vi "aft_xmpl_Shaker Simulation.vi"(8 "error in (no error)":errorcluster, 11 "drive signal":dbl[](array[numeric])) -> (0 "error out":errorcluster, 3 "shaker output":dbl[](array[numeric]))   [LabVIEW 2023]
uses:
  <vilib>/Analysis/3filter.llb/FIR Filter (DBL).vi
  <vilib>/Analysis/NI_AALBase.lvlib
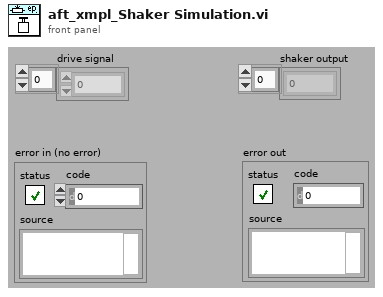
[diagram p1: front panel]
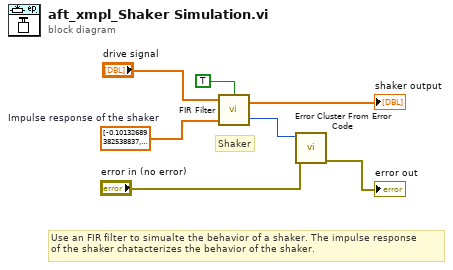
[diagram p0: block diagram]
diagram:
  w5 = dbl[] [-0.10132689382538837, 0.021979664110432052, 0.04315961316267942, 0.010003234659880811, -0.02453838315972942, -0.029502391384022945, -0.01133403262477631, 0.0034751099930438204, 0.0006094985078576808, -0.011755479836677067, 0.001327605245002951, -0.0033771056761639387, 4.464155492825047e-05, 0.006565708408768082, 0.009962874867120263, 0.008639074344455794, 0.0047791927154769865, 0.001573831490921712, 0.001451693602515742, 0.004559921753410905, 0.007887958425535937, 0.007535799875060259, 0.002884203798574461, -0.001344314217800628, 0.0003799233173196481, 0.006770849192730407, 0.008993493616569854, 0.0016727113712982828, -0.0075415788358042584, -0.005082257913402113, 0.009631454746260345, 0.019115298279073174, 0.00975192801362449, -0.006673775899013366, -0.00727738852199998, 0.008282224932711251, 0.0179374280711509, 0.010111721153453304, -0.002837161239050076, -0.005248237495930041, -0.01829337481074023, -0.014559112148119285, -0.00785873219123632, -0.006510188276304974, -0.0112073117350225, -0.017047677712816157, -0.01931329338908274, -0.017522974648444132, -0.01428063109429734, -0.013219572704088585, -0.016207493968072185, -0.022197964957867387, -0.025164751702279345, -0.019917848802463393, -0.010003505438597383, -0.009047112558727675, -0.024502074398267223, -0.04349173301200617, -0.037907672601446694, 0.0005267348932624179, 0.036185298785165985, 0.01294930549478134, -0.07170984775857815, -0.12989866712754808, -0.046243113438134274, 0.1872315514487185, 0.41830304293636617, 0.45467311155623347, 0.2633211894587754, 0.010595653143360029, -0.11994589325572357, -0.09220264292519749, -0.00599216332217202, 0.035633577082091895, 0.015661295308099395, -0.01832802112927939, -0.025735352081092618, -0.008471809884706962, 0.008229490377812898, 0.009524842986507527, 0.001327605245002951, -0.0033771056761639387, 4.464155492825047e-05, 0.006565708408768082, 0.009962874867120263, 0.008639074344455794, 0.0047791927154769865, 0.001573831490921712, 0.001451693602515742, 0.004559921753410905, 0.007887958425535937, 0.007535799875060259, 0.002884203798574461, -0.001344314217800628, 0.0003799233173196481, 0.006770849192730407, 0.008993493616569854, 0.0016727113712982828, -0.0075415788358042584, -0.005082257913402113, 0.009631454746260345, 0.019115298279073174, 0.00975192801362449, -0.006673775899013366, -0.00727738852199998, 0.008282224932711251, 0.0179374280711509, 0.010111721153453304, -0.002837161239050076, -0.005248237495930041, 0.002404488060745071, 0.00887089570481903, 0.007901788010002303, 0.0027392334378310342, -0.0011633868582299584, -0.002088968488861745, -0.0012220546674807486, 0.00036348091969339437, 0.0021901096740054734, 0.0030039949540063425, 0.0012408136005707096, -0.0020922540604038317, -0.00230573461244562, 0.003782641047101538, 0.011413893200078655, 0.00989233225781435, -0.004979323980230643, -0.020788137822369376, -0.011625563465474066, 0.04926146181842194]  # Impulse response of the shaker
  # "Use an FIR filter to simualte the behavior of a shaker. The impulse response\nof the shaker chatacterizes the behavior of the shaker."
  # "Shaker"
  n1 = call-poly <vilib>:"FIR Filter.vi"("init/cont (init:F)"=TRUE, "FIR Coefficients"=w5, "X"="drive signal") -> ("error"=w3:i32, "Filtered X"=→"shaker output":dbl[])  [unwired: 1 in]
  n2 = call <vilib>:"Error Cluster From Error Code.vi"("error in (no error)"="error in (no error)", "error code (0)"=w3) -> ("error out"=→"error out":errorcluster)  [unwired: 1 in, 6 out]
